vi "Insert Bundle by Name - Single Converter.vi"(8 "error in":errorcluster, 11 "vi in":refnum<vi>) -> (0 "error out":errorcluster, 1 "named bundler":refnum<vi>, 2 "wrapper refnum":refnum<vi>)   [LabVIEW 2021, in "Converter.lvlib"]
uses:
  Converter.lvlib
  Path Functions/Path Functions.lvlib
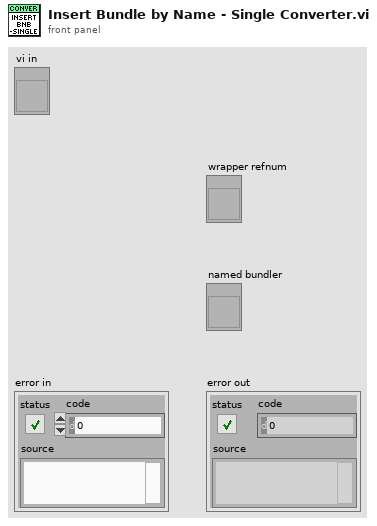
[diagram p1: front panel]
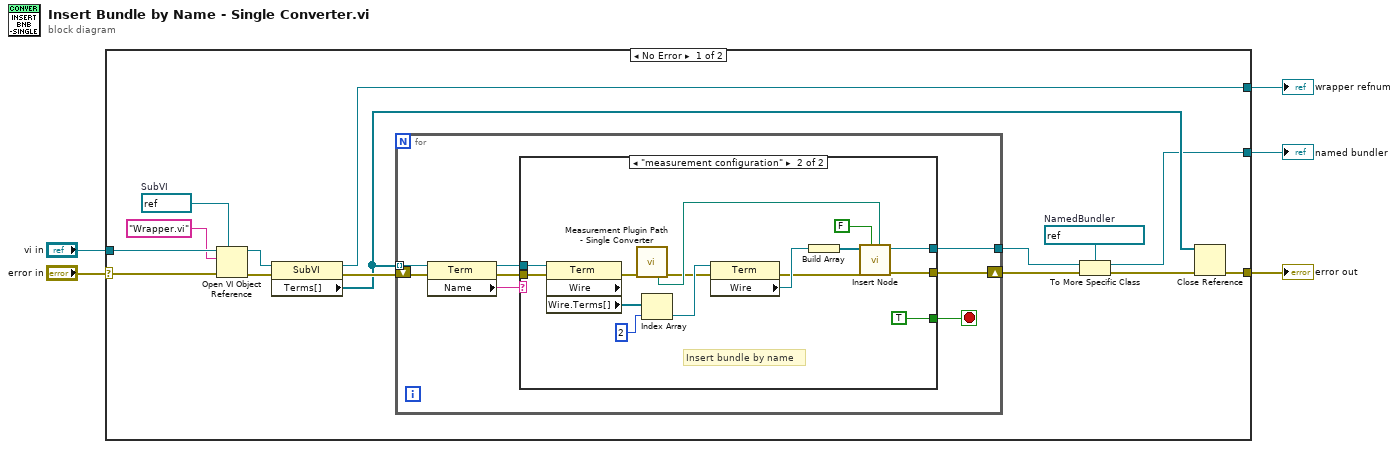
[diagram p0: block diagram]
diagram:
  n1 = case shown="No Error" "error in" {
    selector: "error in" -> [w19 w45]
    tunnel: "vi in" -> [w18 _]
    tunnel: [w13 _] -> w3
    tunnel: [w6 _] -> w2
    tunnel: [w12 w45] -> w1
    frame No Error {
      w8 = refnum<vi> refnum  # NamedBundler
      w20 = refnum<vi> refnum  # SubVI
      n2 = Open VI Object Reference(7:w20, 8:w19, 10:"Wrapper.vi" ("name/order"), 11:w18) -> (0:w15:errorcluster, 3:w17:refnum<vi>)
      n3 = property class="SubVI"(reference=w17, error in=w15) -> (reference out=w13:refnum<vi>, error out=w16:errorcluster, "Terms[]"=w11:refnum<vi>[])
      n4 = for {
        tunnel: w11 -> [w28] mode=indexing
        tunnel: [w23] -> w7
        shift-right: [w24] -> w9
        shift-left: w16 -> [w26]
        stop <- w22 stop-if-true
        n5 = property class="Term"(reference=w28, error in=w26) -> (reference out=w27:refnum<vi>, error out=w25:errorcluster, "Name"=w21:string)
        n6 = case shown="\"measurement configuration\"" w21 {
          tunnel: w27 -> [_ w40]
          tunnel: w25 -> [w29 w44]
          tunnel: [w29 w43] -> w24
          tunnel: [_ w42] -> w23
          tunnel: [_ TRUE] -> w22
          frame Default {
          }
          frame "measurement configuration" {
            # "Insert bundle by name"
            n7 = property class="Term" props=["Wire", "Wire", "Terms[]"](reference=w40, error in=w44) -> (error out=w33:errorcluster, "Wire.Terms[]"=w36:refnum<vi>[])  [unwired: 2 out]
            n8 = call "Measurement Plugin Path - Single Converter.vi"("error in"=w33) -> ("logic vi path"=w32:path, "error out"=w31:errorcluster)  [unwired: 2 in, 11 out]
            n9 = Index Array(array=w36, index=2) -> (element=w35:refnum<vi>)
            n10 = property class="Term"(reference=w35, error in=w31) -> (error out=w30:errorcluster, "Wire"=w39:refnum<vi>)  [unwired: 1 out]
            n11 = Build Array(w39) -> (w37:refnum<vi>[])
            n12 = call "Insert Node.vi"("path to lab view file"=w32, "shift pressed?"=FALSE ("Shift Pressed?"), "error in"=w30, "selection list[]"=w37) -> ("error out"=w43:errorcluster, "element"=w42:refnum<vi>)  [unwired: 5 in, 1 out]
          }
        }
      }
      n13 = To More Specific Class(target class=w8, reference=w7, error in=w9) -> (specific class reference=w6:refnum<vi>, error out=w10:errorcluster)
      n14 = Close Reference(reference=w11, error in (no error)=w10) -> (error out=w12:errorcluster)
    }
    frame Error {
    }
  }
  "error out" <- w1
  "wrapper refnum" <- w3
  "named bundler" <- w2
